vi "Write Range UI.vi"(8 "error in (no error)":errorcluster, 9 "Reader Time":dbl[unit], 10 "Set UI to input? (F)":bool, 11 "Scanner in":refnum<class "Scanner.lvclass">) -> (0 "error out":errorcluster, 3 "Scanner out":refnum<class "Scanner.lvclass">)   [LabVIEW 2015, in "Scanner.lvclass"]
doc: "A Setup UI method for the superclass \"Range\" of scanner."
uses:
  Scanner.lvclass
  Scanner.lvclass/Scanner.ctl
  Range.ctl
panel:
  in  "Return to":dbl
  in  "Return to...?":bool
  out "Time Estimate":string
  out "# Points":u32
  in  "Last":dbl
  in  "Step Size":dbl=1.0 min=0.0
  in  "First":dbl
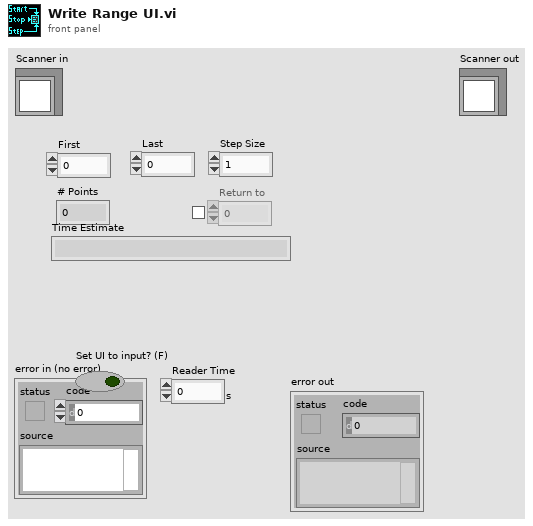
[diagram p1: front panel]
types:
  T1 = typedef "Scanner.lvclass/Range.ctl" = cluster{"xi":dbl, "xf":dbl, "dx":dbl, "Return to...?":bool, "Return to":dbl}
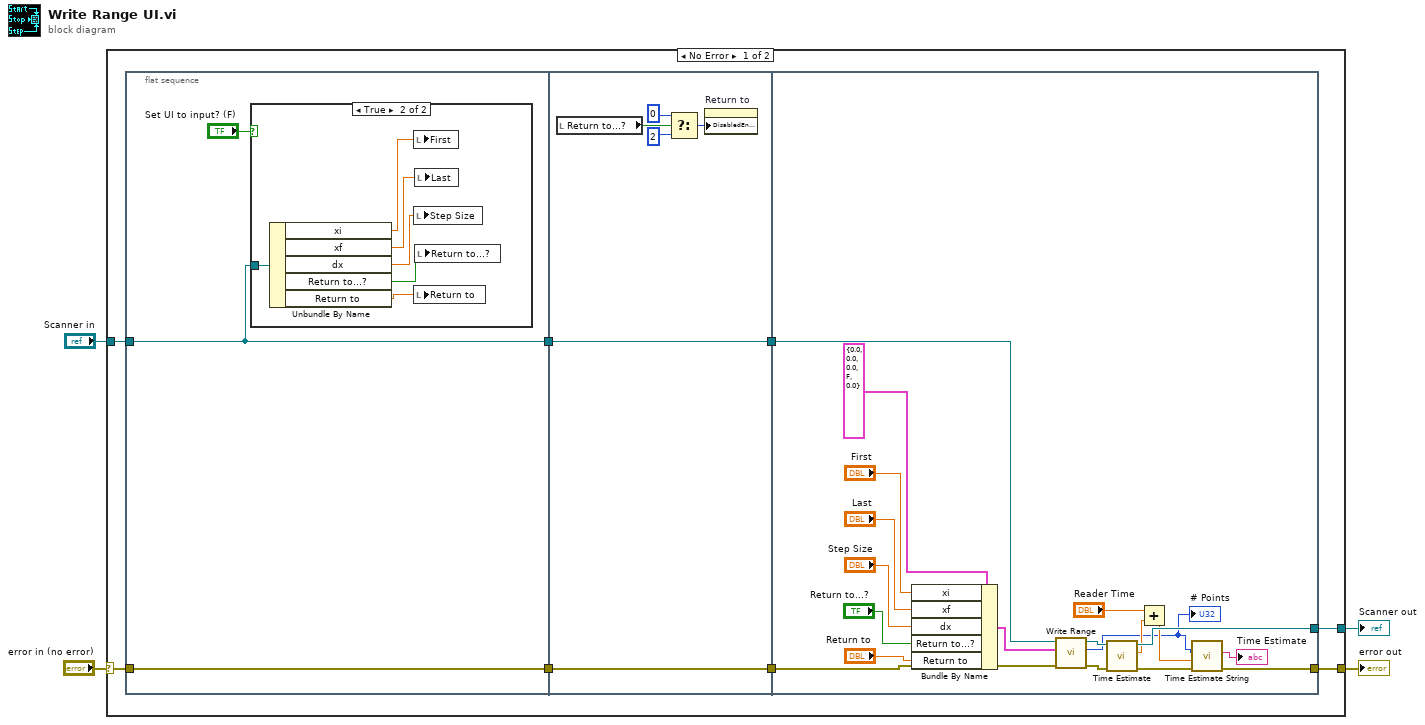
[diagram p0: block diagram]
diagram:
  n1 = case shown="No Error" "error in (no error)" {
    selector: "error in (no error)" -> [w11 w48]
    tunnel: [w9 w48] -> w3
    tunnel: [w10 w47] -> w1
    tunnel: "Scanner in" -> [w12 w47]
    frame No Error {
      n2 = flat-sequence {
        tunnel: w11 -> [w15]
        tunnel: w12 -> [w13]
        tunnel: [w13] -> w8
        tunnel: [w15] -> w6
        tunnel: w8 -> [w27]
        tunnel: [w27] -> w7
        tunnel: w6 -> [w26]
        tunnel: [w26] -> w5
        tunnel: [w45] -> w10
        tunnel: [w28] -> w9
        tunnel: w7 -> [w37]
        tunnel: w5 -> [w46]
        frame #0 {
          n3 = case shown="True" "Set UI to input? (F)" {
            tunnel: w13 -> [_ w21]
            frame False {
            }
            frame True {
              n4 = Unbundle By Name(w21) -> ("xi"=w19:dbl, "xf"=w18:dbl, "dx"=w20:dbl, "Return to...?"=w17:bool, "Return to"=w16:dbl)
              n5 = local write "First"(w19) -> ()
              n6 = local write "Step Size"(w20) -> ()
              n7 = local write "Return to"(w16) -> ()
              n8 = local write "Last"(w18) -> ()
              n9 = local write "Return to...?"(w17) -> ()
            }
          }
        }
        frame #1 {
          n10 = local read "Return to...?"() -> (w24:bool)
          n11 = Select(t=0, s=w24, f=2) -> (s? t:f=w25:i32)
          n12 = property on="Return to" class="DigNum (strict)"("DisabledEnum"=w25) -> ()  [unwired: 2 in, 2 out]
        }
        frame #2 {
          n13 = Bundle By Name(cluster=T1 {"xi"=0.0, "xf"=0.0, "dx"=0.0, "Return to...?"=FALSE, "Return to"=0.0} ("Range"), "xi"="First", "xf"="Last", "dx"="Step Size", "Return to...?"="Return to...?", "Return to"="Return to") -> (w35:T1)
          n14 = call-dynamic "Write Range.vi"("error in (no error)"=w46, "Range"=w35, "Scanner in"=w37) -> ("error out"=w43:errorcluster, "# Points"=w29:u32, "Scanner out"=w44:refnum<class "Scanner.lvclass">)  [unwired: 3 in, 3 out]
          "# Points" <- w29
          n15 = call-dynamic "Time Estimate.vi"("error in (no error)"=w43, "Scanner.lvclass"=w44) -> ("error out"=w32:errorcluster, "time"=w34:dbl[unit], "Scanner.lvclass out"=w45:refnum<class "Scanner.lvclass">)  [unwired: 2 in, 5 out]
          n16 = Add(x="Reader Time", y=w34) -> (x+y=w31:dbl[unit])
          n17 = call "Time Estimate String.vi"("error in (no error)"=w32, "Time"=w31, "Steps"=w29) -> ("error out"=w28:errorcluster, "Time Estimate String"=→"Time Estimate":string)  [unwired: 7 in]
        }
      }
    }
    frame Error {
    }
  }
  "error out" <- w3
  "Scanner out" <- w1
